vi "SetMultiLineColor.vi"(7 "色指定":cluster{"背景色":u32, "文字色":u32}, 8 "Error In":errorcluster caption="エラー入力", 9 "長さ":i32, 10 "開始行":i32, 11 "Tbl refnum":refnum<vi>) -> (0 "Error Out":errorcluster caption="エラー出力", 3 "Tbl refnum出力":refnum<vi>)   [LabVIEW 2014]
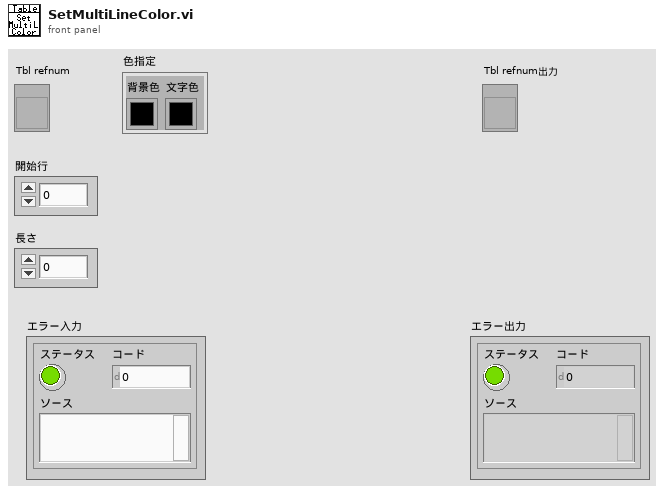
[diagram p1: front panel]
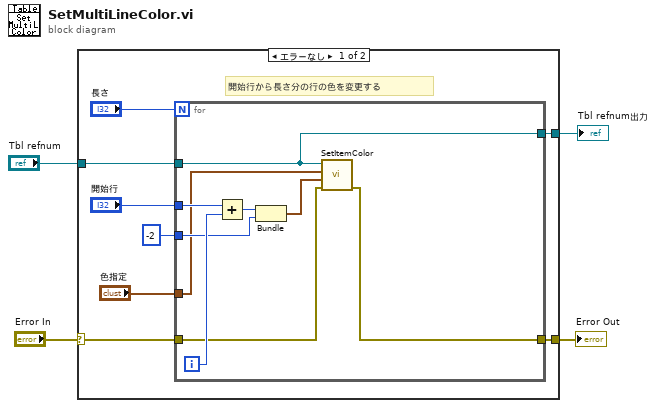
[diagram p0: block diagram]
diagram:
  n1 = case shown="エラーなし" "Error In" {
    selector: "Error In" -> [w8 w23]
    tunnel: [w7 w23] -> w3
    tunnel: "Tbl refnum" -> [w6 w22]
    tunnel: [w5 w22] -> w1
    frame No Error {
      # "開始行から長さ分の行の色を変更する"
      n2 = for {
        N: "長さ" -> [_]
        tunnel: w6 -> [w13]
        tunnel: "開始行" -> [w21]
        tunnel: -2 -> [w18]
        tunnel: "色指定" -> [w16]
        tunnel: w8 -> [w15]
        tunnel: [w14] -> w7
        tunnel: [w13] -> w5
        i -> [w20]
        n3 = Add(x=w21, y=w20) -> (x+y=w19:i32)
        n4 = Bundle(w19, w18) -> (w17:cluster{i32, i32})  [unwired: 1 in]
        n5 = call "SetItemColor.vi"("エラー入力(エラーなし)"=w15, "行列指定"=w17, "色指定"=w16, "Tbl refnum"=w13) -> ("エラー出力"=w14:errorcluster)  [unwired: 7 in]
      }
    }
    frame Error {
    }
  }
  "Error Out" <- w3
  "Tbl refnum出力" <- w1
